vi "IFD_0 Tags.vi"(8 "error in (no error)":errorcluster, 9 "Software Name and Version":string, 10 "System Name":string, 11 "IFD in":refnum<class "IFD.lvclass">) -> (0 "error out":errorcluster, 3 "IFD out":refnum<class "IFD.lvclass">)   [LabVIEW 2016, in "IFD.lvclass"]
uses:
  IFD.lvclass
  Tag/IFD_Tag.lvclass/IFD_Tag.ctl
  IFD.lvclass/IFD.ctl
  Tag/IFD_Tag.lvclass
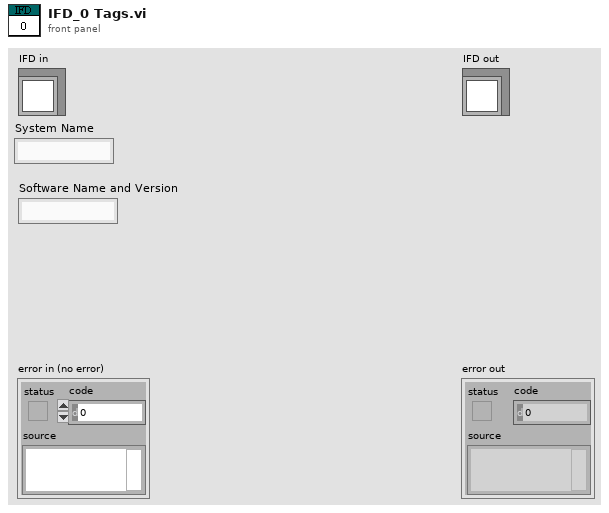
[diagram p1: front panel]
types:
  T1 = enum16{"big-endian, network order", "native, host order", "little-endian"}
  T2 = enum16{"Undefined(DO NOT USE)", "U8", "ASCII", "U16", "U32", "RATIONAL", "I8", "Undefined 8 bit", "I16", "I32", "SRATIONAL", "SGL", "DBL"}
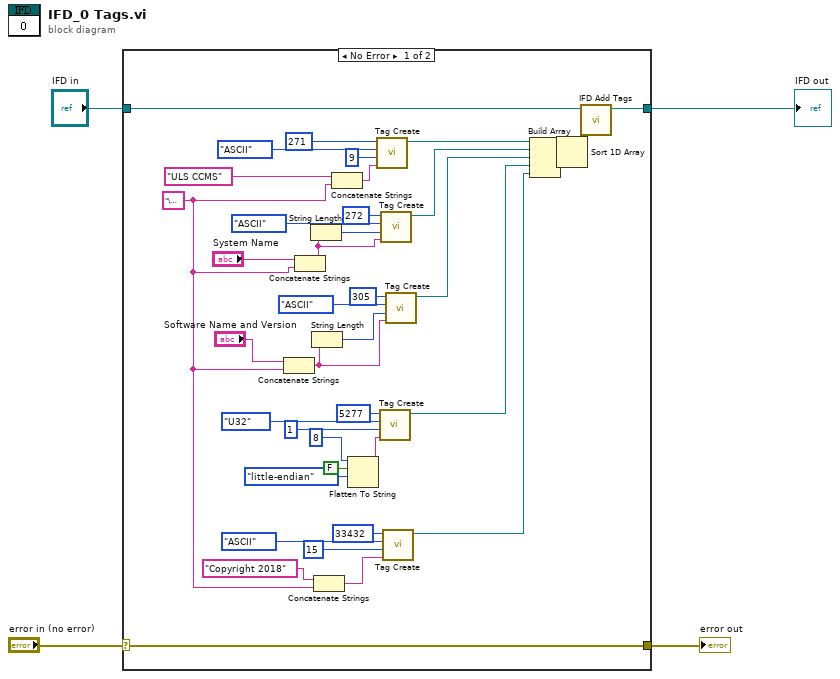
[diagram p0: block diagram]
diagram:
  n1 = case shown="No Error" "error in (no error)" {
    selector: "error in (no error)" -> [w42 w44]
    tunnel: [w42 w44] -> w3
    tunnel: [w40 w43] -> w1
    tunnel: "IFD in" -> [w41 w43]
    frame No Error {
      w14 = "\u0000"
      n2 = Concatenate Strings("Software Name and Version", w14) -> (w21:string)
      n3 = Concatenate Strings("System Name", w14) -> (w26:string)
      n4 = String Length(string=w26) -> (length=w27:i32)
      n5 = String Length(string=w21) -> (length=w22:i32)
      n6 = Concatenate Strings("Copyright 2018", w14) -> (w13:string)
      n7 = Concatenate Strings("ULS CCMS", w14) -> (w31:string)
      n8 = Flatten To String(anything=u32 8, prepend array or string size? (T)=FALSE, byte order (0:big-endian, network order)=T1."little-endian") -> (data string=w7:string)  [unwired: 1 in, 2 out]
      n9 = call "Tag Create.vi"("Data"=w31, "Data Count"=u32 9, "Data Type"=T2."ASCII", "Tag ID"=u16 271) -> ("IFD_Tag out"=w39:refnum<class "IFD_Tag.lvclass">)  [unwired: 7 in]
      n10 = call "Tag Create.vi"("Data"=w7, "Data Count"=u32 1, "Data Type"=T2."U32", "Tag ID"=u16 5277) -> ("IFD_Tag out"=w10:refnum<class "IFD_Tag.lvclass">)  [unwired: 7 in]
      n11 = call "Tag Create.vi"("Data"=w26, "Data Count"=w27, "Data Type"=T2."ASCII", "Tag ID"=u16 272) -> ("IFD_Tag out"=w37:refnum<class "IFD_Tag.lvclass">)  [unwired: 7 in]
      n12 = call "Tag Create.vi"("Data"=w13, "Data Count"=u32 15, "Data Type"=T2."ASCII", "Tag ID"=u16 33432) -> ("IFD_Tag out"=w11:refnum<class "IFD_Tag.lvclass">)  [unwired: 7 in]
      n13 = call "Tag Create.vi"("Data"=w21, "Data Count"=w22, "Data Type"=T2."ASCII", "Tag ID"=u16 305) -> ("IFD_Tag out"=w36:refnum<class "IFD_Tag.lvclass">)  [unwired: 7 in]
      n14 = Build Array(w39, w37, w36, w10, w11) -> (w38:refnum<class "IFD_Tag.lvclass">[])
      n15 = Sort 1D Array(array=w38) -> (sorted array=w9:refnum<class "IFD_Tag.lvclass">[])
      n16 = call "IFD Add Tags.vi"("Tag(s)"=w9, "IFD in"=w41) -> ("IFD out"=w40:refnum<class "IFD.lvclass">)  [unwired: 8 in, 1 out]
    }
    frame Error {
    }
  }
  "error out" <- w3
  "IFD out" <- w1
